vi "MU Mt Sync Analyze Data.vi"(8 "error in (no error)":errorcluster, 9 "numberOfSamples":u64, 10 "data":T1(array[cluster]), 11 "mtSyncHandle":T3) -> (0 "error out":errorcluster, 3 "mtSyncAnalyzeResultHandle":T2)   [LabVIEW 2017, in "MU_3SL_interface.lvlib"]
uses:
  MU_3SL_interface.lvlib
  handles/mtSyncHandle.ctl
  handles/mtSyncAnalyzeResultHandle.ctl
  lib/MU_3SL_interface.dll
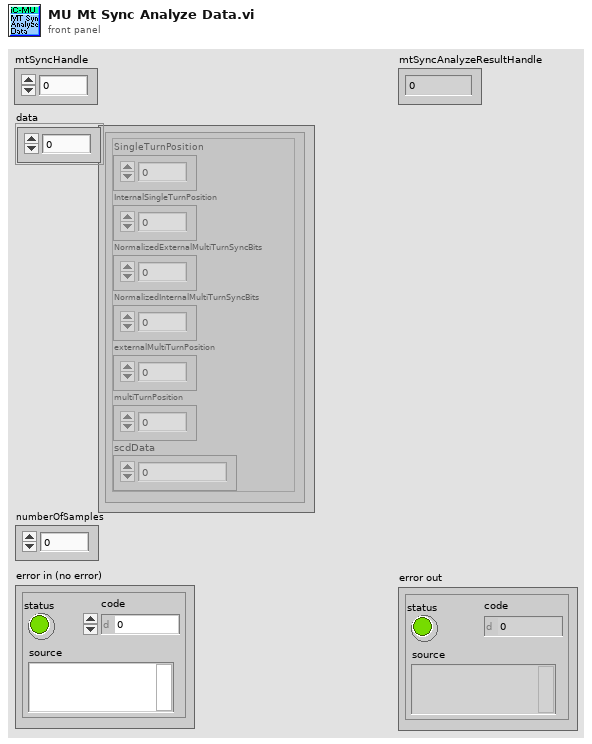
[diagram p1: front panel]
types:
  T1 = cluster{"SingleTurnPosition":u32, "InternalSingleTurnPosition":u32, "NormalizedExternalMultiTurnSyncBits":u32, "NormalizedInternalMultiTurnSyncBits":u32, "externalMultiTurnPosition":u32, "multiTurnPosition":u32, "scdData":u64}[]
  T2 = typedef "MU_3SL_interface.lvlib/mtSyncAnalyzeResultHandle.ctl" = u64
  T3 = typedef "MU_3SL_interface.lvlib/mtSyncHandle.ctl" = u64
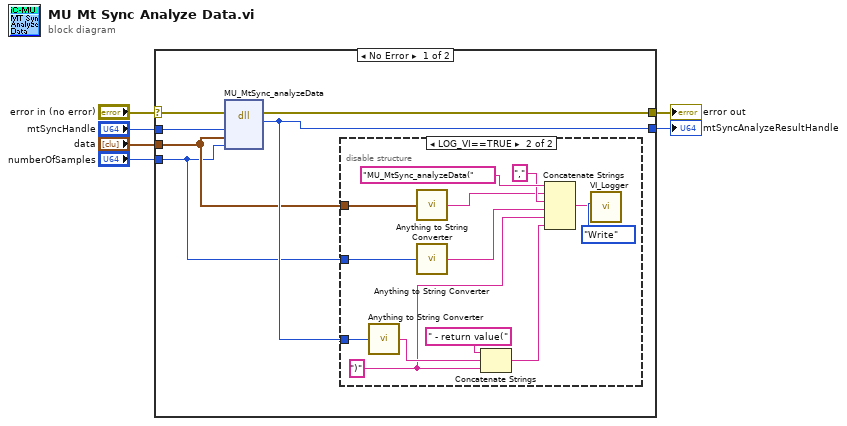
[diagram p0: block diagram]
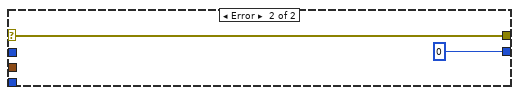
[diagram p3: hidden frame]
diagram:
  n1 = case shown="No Error" "error in (no error)" {
    selector: "error in (no error)" -> [w12 w27]
    tunnel: [w11 u64 0 ("mtSynchHandle")] -> w3
    tunnel: [w10 w27] -> w6
    tunnel: "mtSyncHandle" -> [w9 _]
    tunnel: "data" -> [w8 _]
    tunnel: "numberOfSamples" -> [w7 _]
    frame No Error {
      n2 = dll-call lib="C:/Users/bes/AppData/Roaming/work/mu_9so/icsubmodules/soft_mu_3sl_master/lv_interface/lib/MU_3SL_interface**.*" fn="MU_MtSync_analyzeData"(error in=w12, "mtSynchHandle"=w9, "SynchronisationData"=w8, "numberOfSamples"=w7) -> (error out=w10:errorcluster, "mtSyncAnalyzeResultHandle"=w11:u64)  [unwired: 5 in, 1 out]
      n3 = disable-structure shown="LOG_VI==TRUE" {
        disable-tunnel: w11 -> [_ w20]
        disable-tunnel: w8 -> [_ w14]
        disable-tunnel: w7 -> [_ w18]
        frame condition #0 {
        }
        frame condition #1 (active) {
          w16 = ")" ("string")
          n4 = call "Anything to String Converter.vi"("anything"=w20) -> ("String"=w19:string)
          n5 = call "Anything to String Converter.vi"("anything"=w14) -> ("String"=w13:string)
          n6 = call "Anything to String Converter.vi"("anything"=w18) -> ("String"=w17:string)
          n7 = Concatenate Strings(" - return value(" ("string"), w19, w16) -> (w15:string)
          n8 = Concatenate Strings("MU_MtSync_analyzeData(" ("Info in"), w13, "," ("string"), w17, w16, w15) -> (w23:string)
          n9 = call "VI_Logger.vi"("Action (Read)"=enum16{"Write", "Read"}."Write", "Info in"=w23) -> ()  [unwired: 8 in, 2 out]
        }
      }
    }
    frame Error {
    }
  }
  "error out" <- w6
  "mtSyncAnalyzeResultHandle" <- w3
